vi "Ping core.vi"(8 "error in (no error)":errorcluster, 10 "Emission":T1, 11 "UI_Actor in":refnum<class "UI_Actor.lvclass">) -> (0 "error out":errorcluster, 3 "UI_Actor out":refnum<class "UI_Actor.lvclass">)   [LabVIEW 2020, in "UI_Actor.lvlib" / "UI_Actor.lvclass"]
uses:
  UI_Actor.lvclass
  D:/Projets/STEP AT/UI Actor/support/Actor Framework.lvlibp/1abvi3w/vi.lib/ActorFramework/Actor/Actor.lvclass
  ctl_Ping payload.ctl
  UI_Actor.lvclass/UI_Actor.ctl
  UI_Actor Messages/Ping core Msg/Ping core Msg.lvclass/Ping core Msg.ctl
  UI_Actor Messages/Ping return Msg/Ping return Msg.lvclass/Ping return Msg.ctl
  Read Name.vi
  support/Actor Framework.lvlibp/1abvi3w/vi.lib/ActorFramework/Message Enqueuer/Enqueue.vi
  UI_Actor Messages/Ping core Msg/Ping core Msg.lvclass
  UI_Actor Messages/Ping return Msg/Ping return Msg.lvclass
  support/Actor Framework.lvlibp/1abvi3w/vi.lib/ActorFramework/Actor/Actor.lvclass
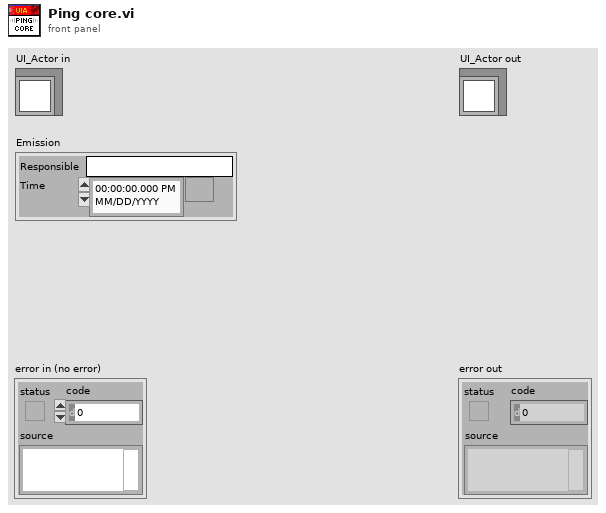
[diagram p1: front panel]
types:
  T1 = typedef "UI_Actor.lvlib/UI_Actor.lvclass/ctl_Ping payload.ctl" = cluster{"Responsible":string, "Time":timestamp}
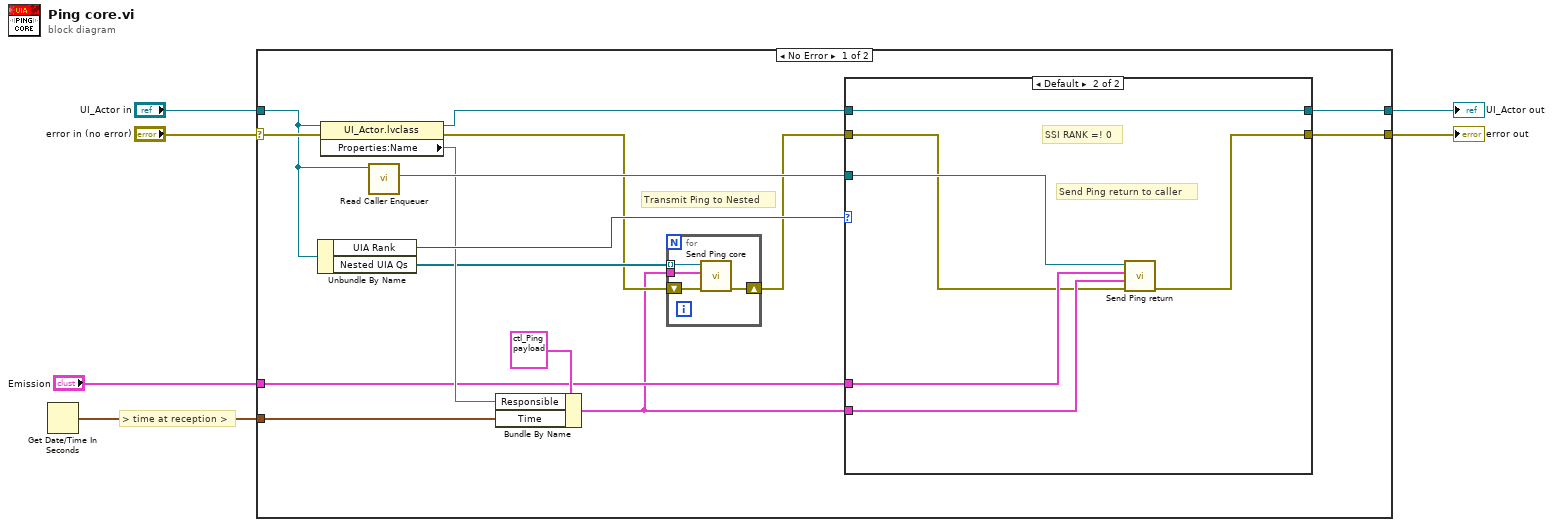
[diagram p0: block diagram]
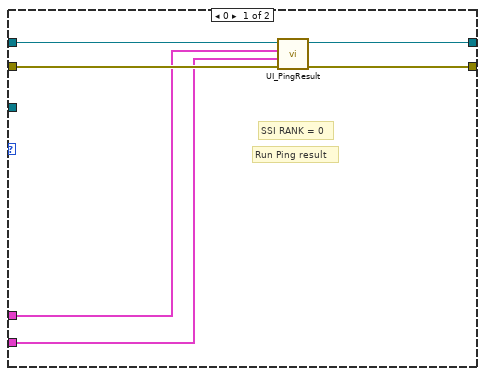
[diagram p2: hidden frame]
diagram:
  # "> time at reception >"
  n1 = Get Date/Time In Seconds() -> (seconds since 1Jan1904=w2:timestamp)
  n2 = case shown="No Error" "error in (no error)" {
    selector: "error in (no error)" -> [w21 w39]
    tunnel: [w20 w39] -> w5
    tunnel: [w16 w38] -> w3
    tunnel: "UI_Actor in" -> [w17 w38]
    tunnel: w2 -> [w12 _]
    tunnel: "Emission" -> [w10 _]
    frame No Error {
      # "Transmit Ping to Nested"
      n3 = Unbundle By Name(w17) -> ("UIA Rank"=w19:i32, "Nested UIA Qs"=w11:refnum<class "Message Enqueuer.lvclass">[])
      n4 = property class="UI_Actor.lvclass"(reference=w17, error in=w21) -> (reference out=w15:refnum<class "UI_Actor.lvclass">, error out=w9:errorcluster, "Properties:Name"=w13:string)
      n5 = call "Read Caller Enqueuer.vi"("Actor"=w17) -> ("Caller Enqueuer"=w18:refnum<class "Message Enqueuer.lvclass">)  [unwired: 10 in]
      n6 = Bundle By Name(cluster=T1 {"Responsible"="", "Time"=timestamp(0 s since 1904-01-01)} ("Reception"), "Responsible"=w13, "Time"=w12) -> (w7:T1)
      n7 = for {
        tunnel: w11 -> [w25] mode=indexing
        shift-right: [w23] -> w8
        shift-left: w9 -> [w24]
        tunnel: w7 -> [w22]
        n8 = call "Send Ping core.vi"("error in (no error)"=w24, "Emission"=w22, "Message Enqueuer"=w25) -> ("error out"=w23:errorcluster)  [unwired: 7 in, 1 out]
      }
      n9 = case shown="Default" w19 {
        tunnel: w8 -> [w30 w32]
        tunnel: [w29 w35] -> w20
        tunnel: w10 -> [w27 w36]
        tunnel: w18 -> [_ w37]
        tunnel: w15 -> [w31 w34]
        tunnel: [w28 w34] -> w16
        tunnel: w7 -> [w26 w33]
        frame 0 {
          # "SSI RANK = 0"
          # "Run Ping result"
          n10 = call-dynamic "UI_PingResult.vi"("error in (no error)"=w30, "Reception"=w26, "Emission"=w27, "UI_Actor in"=w31) -> ("error out"=w29:errorcluster, "UI_Actor out"=w28:refnum<class "UI_Actor.lvclass">)  [unwired: 6 in]
        }
        frame Default {
          # "Send Ping return to caller"
          # "SSI RANK =! 0"
          n11 = call "Send Ping return.vi"("error in (no error)"=w32, "Reception"=w33, "Emission"=w36, "Message Enqueuer"=w37) -> ("error out"=w35:errorcluster)  [unwired: 6 in, 1 out]
        }
      }
    }
    frame Error {
    }
  }
  "error out" <- w5
  "UI_Actor out" <- w3
